vi "Execute.vi"(8 "error in (no error)":errorcluster, 9 "Consumer Queues in":T1, 10 "UI Process Command in":refnum<class "Init UI Process.lvclass">, 11 "UI Process Data in":T2) -> (0 "error out":errorcluster, 1 "Consumer Queues out":T1, 2 "Stop?":bool, 3 "UI Process Data out":T2)   [LabVIEW 2019, in "User Interface Process.lvlib" / "Init UI Process.lvclass"]
uses:
  Init UI Process.lvclass
  UI Process Data.ctl
  TS Framework/ExeLogging/UI Logger/UI Logger.lvclass
  UI State.ctl
  TS Framework/Consumer Queues.ctl
  Generic UI Command/Generic UI Process Command.lvclass
  DAC Process/Generic DAC Command/Generic DAC Process Command.lvclass
  Trig Process/Generic Trig Command/Generic Trig Process Command.lvclass
  DAC Process/Init DAC Process/Init DAC Process.lvclass
  UI Idle State/UI Idle State.lvclass
  Init UI Process.lvclass/Init UI Process.ctl
  Generic Test Stand/Generic Test Stand.lvclass/Generic Test Stand.ctl
  DAC Process/Init DAC Process/Init DAC Process.lvclass/Init DAC Process.ctl
  Generic Test Stand/Generic Test Stand.lvclass
  User Interface Process.lvlib
  TS Framework/TS Framework.lvlib
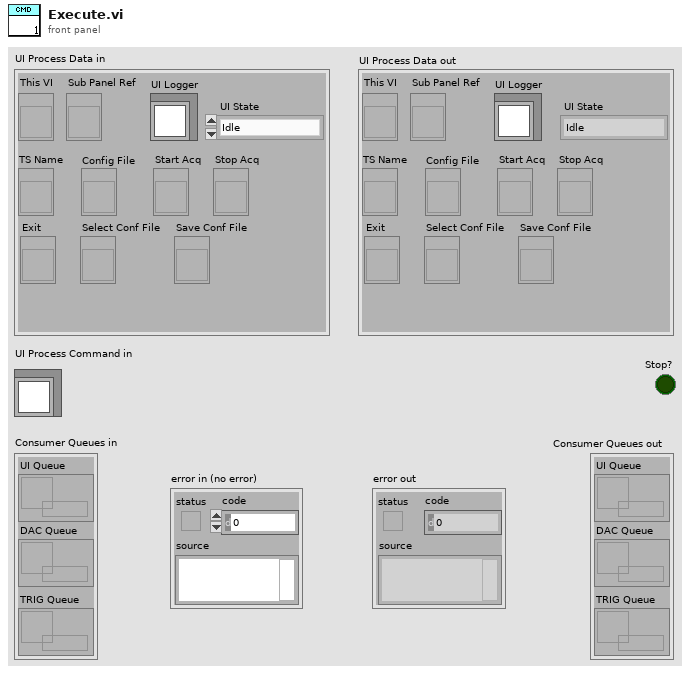
[diagram p1: front panel]
types:
  T1 = typedef "TS Framework.lvlib/Consumer Queues.ctl" = cluster{"UI Queue":refnum<queue>, "DAC Queue":refnum<queue>, "TRIG Queue":refnum<queue>}
  T2 = typedef "User Interface Process.lvlib/UI Process Data.ctl" = cluster{"This VI":refnum<vi>, "Sub Panel Ref":refnum<vi>, "UI Logger":refnum<class "UI Logger.lvclass">, "TS Name":refnum<vi>, "Config File":refnum<vi>, "Start Acq":refnum<vi>, "Stop Acq":refnum<vi>, "Exit":refnum<vi>, "Select Conf File":refnum<vi>, "Save Conf File":refnum<vi>, "UI State":T3}
  T3 = typedef "User Interface Process.lvlib/UI State.ctl" = enum16{"Idle", "Acquiring"}
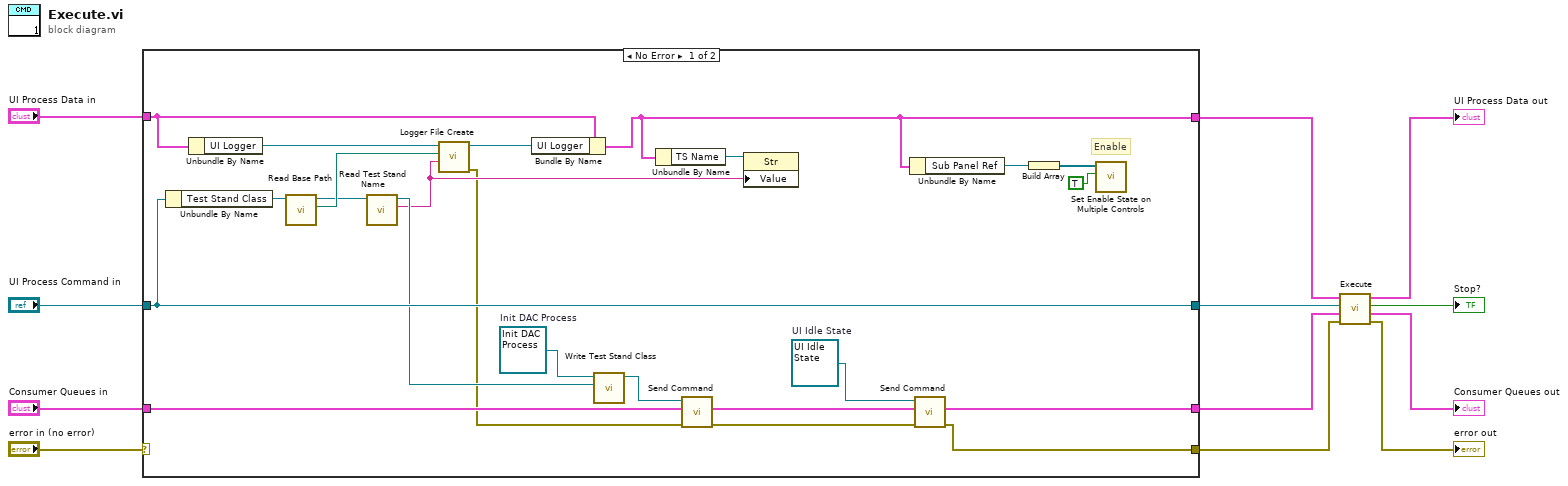
[diagram p0: block diagram]
diagram:
  n1 = case shown="No Error" "error in (no error)" {
    selector: "error in (no error)" -> [_ w38]
    tunnel: "UI Process Command in" -> [w26 w37]
    tunnel: "Consumer Queues in" -> [w34 w36]
    tunnel: [w20 w36] -> w4
    tunnel: "UI Process Data in" -> [w30 w39]
    tunnel: [w14 w39] -> w2
    tunnel: [w17 w38] -> w5
    tunnel: [w26 w37] -> w3
    frame No Error {
      w19 = refnum<class "UI Idle State.lvclass"> refnum  # UI Idle State
      w25 = refnum<class "Init DAC Process.lvclass"> refnum  # Init DAC Process
      # "Enable"
      n2 = Unbundle By Name(w26) -> ("Test Stand Class"=w29:refnum<class "Generic Test Stand.lvclass">)
      n3 = Unbundle By Name(w30) -> ("UI Logger"=w33:refnum<class "UI Logger.lvclass">)
      n4 = call "Read Base Path.vi"("Generic Test Stand in"=w29) -> ("Base Path"=w32:path, "Generic Test Stand out"=w27:refnum<class "Generic Test Stand.lvclass">)  [unwired: 8 in, 1 out]
      n5 = call "Read Test Stand Name.vi"("Generic Test Stand in"=w27) -> ("Test Stand Name"=w23:string, "Generic Test Stand out"=w24:refnum<class "Generic Test Stand.lvclass">)  [unwired: 8 in, 1 out]
      n6 = call-dynamic "Logger File Create.vi"("Test Stand Name"=w23, "Project Base Path"=w32, "UI Logger in"=w33) -> ("error out"=w22:errorcluster, "UI Logger out"=w31:refnum<class "UI Logger.lvclass">)  [unwired: 7 in]
      n7 = Bundle By Name(cluster=w30, "UI Logger"=w31) -> (w14:T2)
      n8 = call "Write Test Stand Class.vi"("Generic Test Stand"=w24, "Init DAC Process in"=w25) -> ("Init DAC Process out"=w35:refnum<class "Init DAC Process.lvclass">)  [unwired: 8 in, 1 out]
      n9 = Unbundle By Name(w14) -> ("TS Name"=w28:refnum<vi>)
      n10 = call-dynamic "Send Command.vi"("error in (no error)"=w22, "Consumer Queues in"=w34, "DAC Process Command"=w35) -> ("error out"=w18:errorcluster, "Consumer Queues out"=w21:T1)  [unwired: 7 in]
      n11 = property class="Str"(reference=w28, "Value"=w23) -> ()  [unwired: 1 in, 2 out]
      n12 = Unbundle By Name(w14) -> ("Sub Panel Ref"=w13:refnum<vi>)
      n13 = call-dynamic "Send Command.vi"("error in (no error)"=w18, "Consumer Queues in"=w21, "UI Process Command in"=w19) -> ("error out"=w17:errorcluster, "Consumer Queues out"=w20:T1)  [unwired: 7 in]
      n14 = Build Array(w13) -> (w15:refnum<vi>[])
      n15 = call "Set Enable State on Multiple Controls.vi"("Enable?"=TRUE, "Controls"=w15) -> ()  [unwired: 10 in]
    }
    frame Error {
    }
  }
  n16 = call-parent "Execute.vi"("error in (no error)"=w5, "Consumer Queues in"=w4, "UI Process Command in"=w3, "UI Process Data in"=w2) -> ("error out"=→"error out":errorcluster, "Consumer Queues out"=→"Consumer Queues out":T1, "Stop?"=→"Stop?":bool, "UI Process Data out"=→"UI Process Data out":T2)  [unwired: 4 in]
